vi "DN4_ContinueCompare_SetCompareTable_Ex.vi"(2 "compare table":i32[][](array[numeric]), 3 "error in (no error)":errorcluster, 4 "Task ID":u32) -> (0 "error out":errorcluster, 1 "Task ID out":u32)   [LabVIEW 2009]
uses:
  Windows/System32/AdvLvDaq.dll
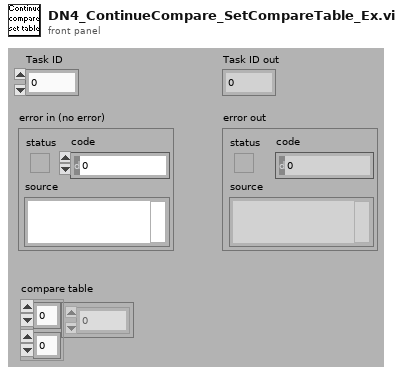
[diagram p1: front panel]
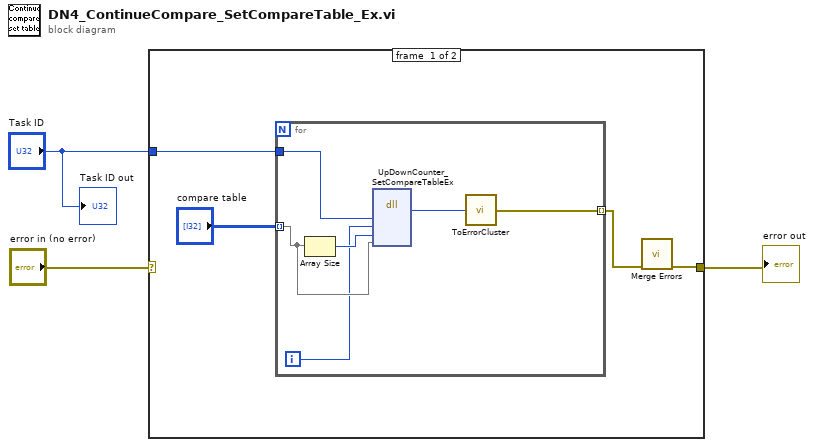
[diagram p0: block diagram]
diagram:
  n1 = case shown="Error" "error in (no error)" {
    selector: "error in (no error)" -> [_ w14]
    tunnel: "Task ID" -> [w7 _]
    tunnel: [w4 w14] -> w1
    frame #0 {
      n2 = for {
        tunnel: w7 -> [w13]
        tunnel: [w11] -> w5 mode=indexing
        tunnel: "compare table" -> [w9] mode=indexing
        i -> [w8]
        n3 = Array Size(array=w9) -> (size(s)=w10:i32)
        n4 = dll-call lib="C:/Windows/System32/AdvLvDaq.dll" fn="UpDownCounter_SetCompareTableEx"("taskID"=w13, "channelIndex"=w8, "tableSize"=w10, "table"=w9) -> ("return type"=w12:i32)  [unwired: 6 in, 3 out]
        n5 = call <userlib>:"ToErrorCluster.vi"("error code"=w12) -> ("error out"=w11:errorcluster)
      }
      n6 = call <vilib>:"Merge Errors.vi"("error array in"=w5) -> ("error out"=w4:errorcluster)  [unwired: 3 in, 3 out]
    }
    frame #1 {
    }
  }
  "error out" <- w1
  "Task ID out" <- "Task ID"
